vi "ADQ Create ADQ Control Unit (ILYA).vi"(8 "error in (no error)":errorcluster) -> (0 "error out":errorcluster, 3 "function return":u32)   [LabVIEW 2013]
doc: "extern \"C\" __declspec(dllimport) void* CreateADQControlUnit();"
uses:
  dlls/ADQAPI.dll
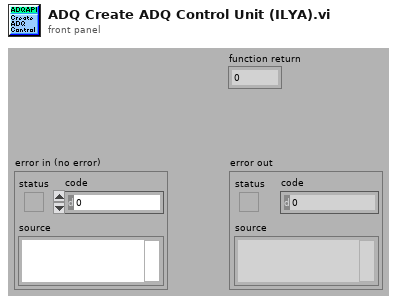
[diagram p1: front panel]
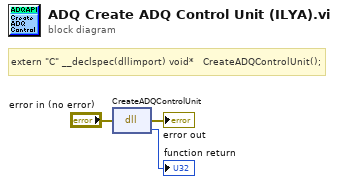
[diagram p0: block diagram]
diagram:
  # "extern \"C\" __declspec(dllimport) void*\t\t\tCreateADQControlUnit();"
  n1 = dll-call lib="C:/Users/astafiev/Desktop/IlyaDrive/@photonCounting/LabView_Imperium/dlls/ADQAPI.*" fn="CreateADQControlUnit"(error in="error in (no error)") -> (error out=→"error out":errorcluster, "return type"=→"function return":u32)  [unwired: 2 in, 1 out]
